vi "4.调用百度地图API.vi"(0 "WebBrowser":refnum<k7>(container), 1 "?":dbl(slide) scale=5.0..15.0) -> ()   [LabVIEW 2018]
panel:
  in  "?":bool
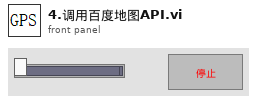
[diagram p1: front panel]
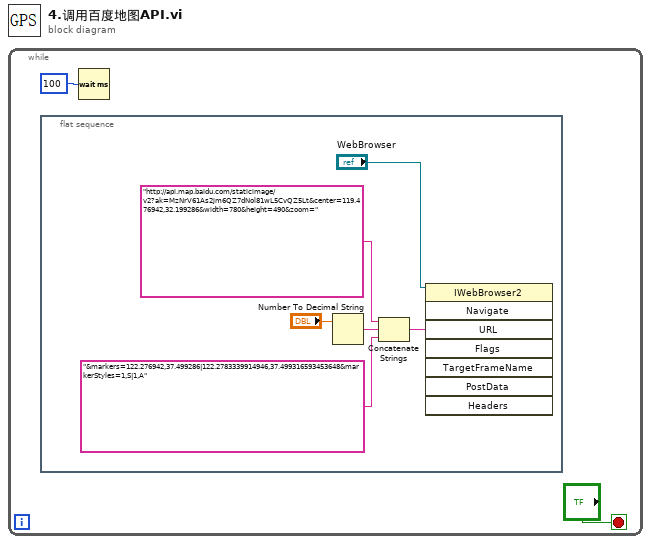
[diagram p0: block diagram]
diagram:
  n1 = while {
    stop <- "?" stop-if-true
    n2 = flat-sequence {
      frame #0 {
        n3 = Number To Decimal String(number="?") -> (decimal integer string=w5:string)  [unwired: 1 in]
        n4 = Concatenate Strings("http://api.map.baidu.com/staticimage/v2?ak=MzNrV61As2jm6QZ7dNol81wL5CvQZ5Lt&center=119.476942,32.199286&width=780&height=490&zoom=", w5, "&markers=122.276942,37.499286|122.2783339914946,37.499316593453648&markerStyles=1,S|1,A") -> (w3:string)
        n5 = invoke class="IWebBrowser2" method="Navigate"(reference="WebBrowser", "URL"=w3) -> ()  [unwired: 6 in, 8 out]
      }
    }
    n6 = Wait (ms)(milliseconds to wait=u32 100 ("等待时间（毫秒）")) -> ()  [unwired: 1 out]
  }
